vi "Destroy.vi"(8 "error in":errorcluster, 11 "Gantry Class in":refnum<class "Gantry.lvclass">) -> (0 "error out":errorcluster)   [LabVIEW 2017, in "Gantry.lvclass"]
uses:
  Gantry.lvclass
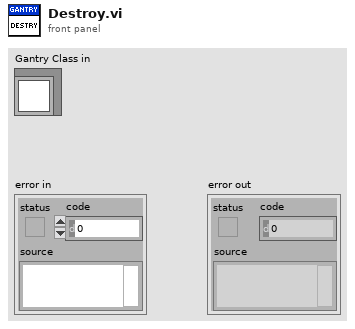
[diagram p1: front panel]
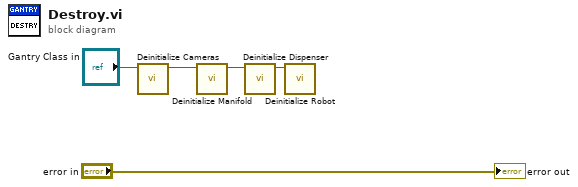
[diagram p0: block diagram]
diagram:
  n1 = call-dynamic "Deinitialize Cameras.vi"("Gantry in"="Gantry Class in") -> ("Gantry out"=w2:refnum<class "Gantry.lvclass">)  [unwired: 9 in, 1 out]
  n2 = call-dynamic "Deinitialize Manifold.vi"("Gantry Class in"=w2) -> ("Gantry Class out"=w3:refnum<class "Gantry.lvclass">)  [unwired: 9 in, 1 out]
  n3 = call-dynamic "Deinitialize Dispenser.vi"("Gantry Class in"=w3) -> ("Gantry Class out"=w1:refnum<class "Gantry.lvclass">)  [unwired: 9 in, 1 out]
  n4 = call-dynamic "Deinitialize Robot.vi"("Gantry in"=w1) -> ()  [unwired: 9 in, 2 out]
  "error out" <- "error in"
